vi "Test Timer Module API.vi"() -> ()   [LabVIEW 2018]
doc: "Timer Module API Tester."
uses:
  Timer Module.lvlib
panel:
  out "Timers":timestamp[](array[timestamp]) format="%^<%H:%M:%S%3u>T"
  in  "Pause Timer":bool
  in  "Start/Reset Timer":bool
  in  "Run as Singleton?":bool
  in  "Show Block Diagram":bool
  in  "Refresh Modules":bool
  out "Active Modules":string[](array[string])
  in  "Stop Module":bool
  in  "Select Module":i32(ring)=-1 caption="Select Module\nTo send Request to" items=["All"=-1]
  in  "Run New Module":bool
  in  "Hide Module Panel":bool
  in  "Show Module Panel":bool
  out "Status":string
  # "This VI tests the API for the Module."
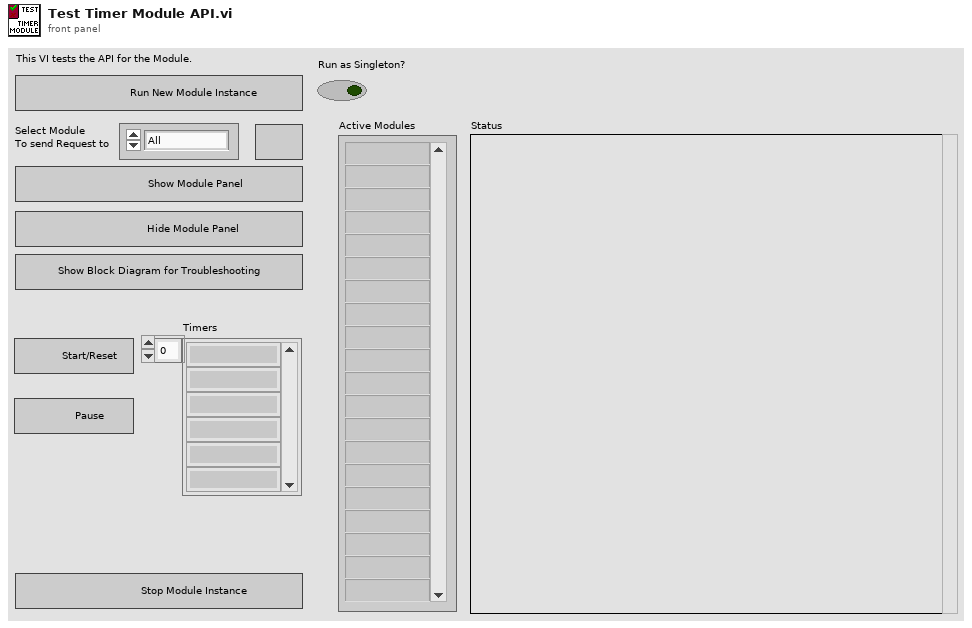
[diagram p1: front panel]
types:
  T1 = typedef "Timer Module.lvlib/Broadcast Events--cluster.ctl" = cluster{"Module Did Init":refnum<user-event>, "Status Updated":refnum<user-event>, "Error Reported":refnum<user-event>, "Module Did Stop":refnum<user-event>, "Update Module Execution Status":refnum<user-event>, "Timer Updated":refnum<user-event>}
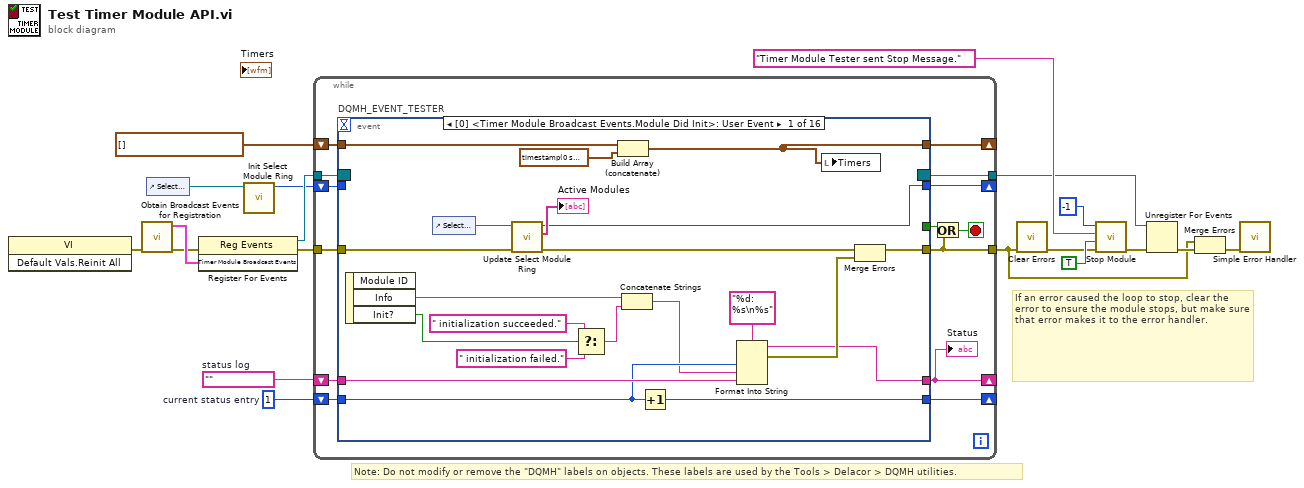
[diagram p0: block diagram]
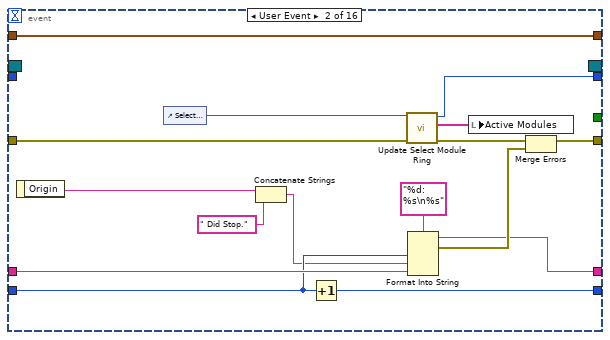
[diagram p2: hidden frame]
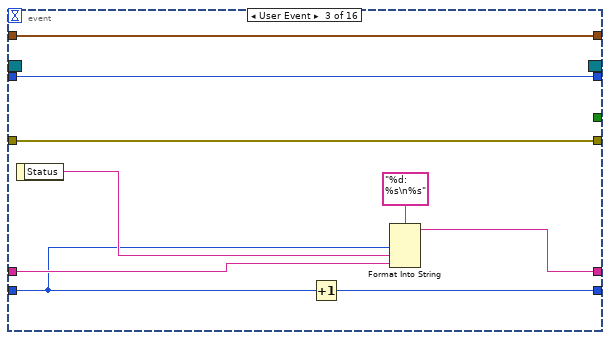
[diagram p3: hidden frame]
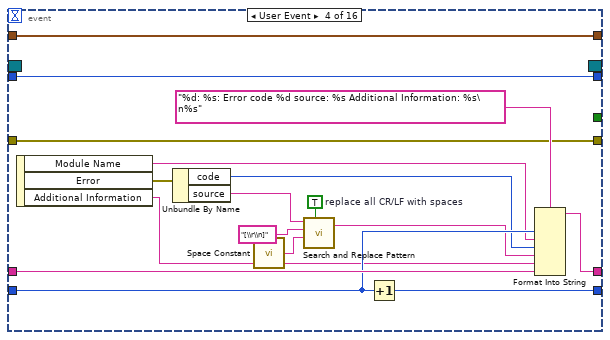
[diagram p4: hidden frame]
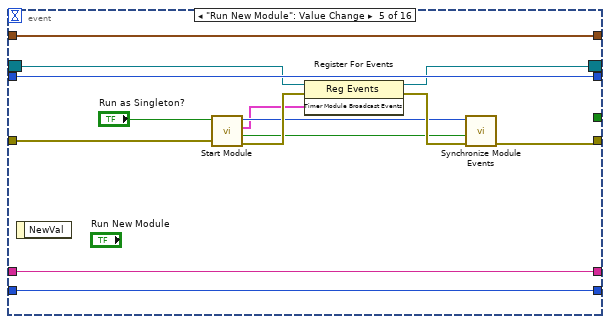
[diagram p5: hidden frame]
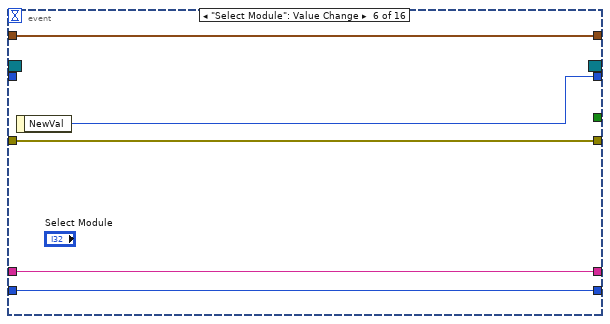
[diagram p6: hidden frame]
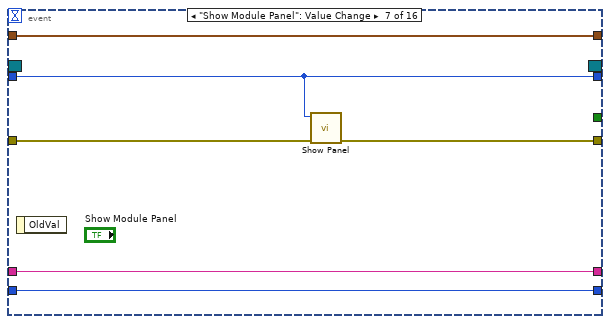
[diagram p7: hidden frame]
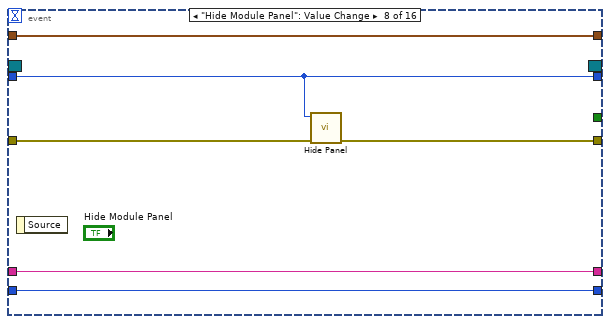
[diagram p8: hidden frame]
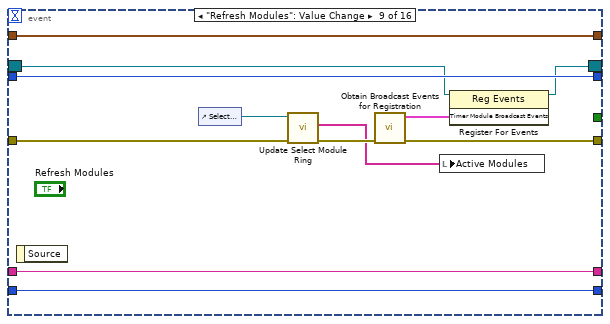
[diagram p9: hidden frame]
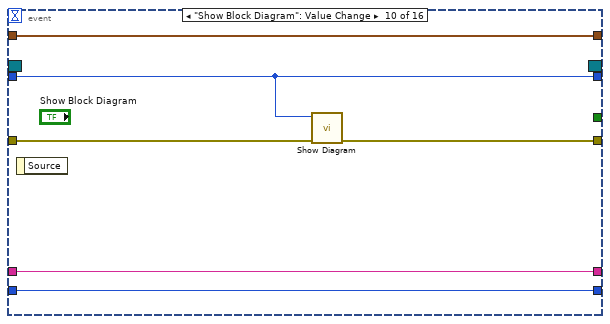
[diagram p10: hidden frame]
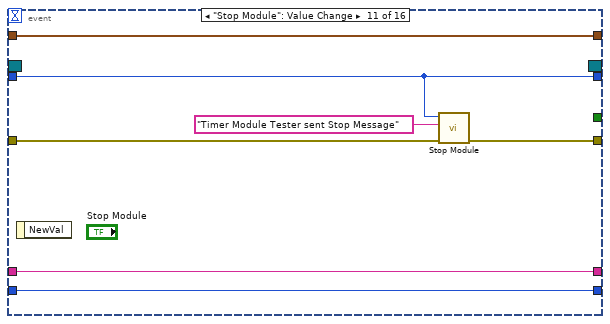
[diagram p11: hidden frame]
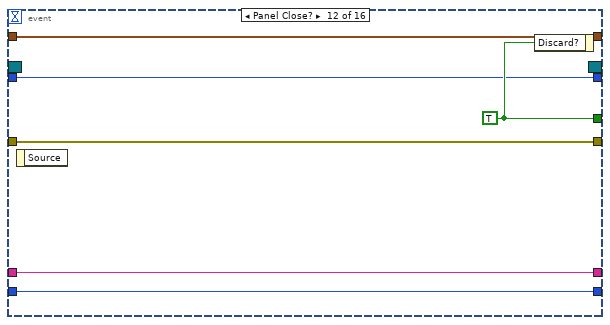
[diagram p12: hidden frame]
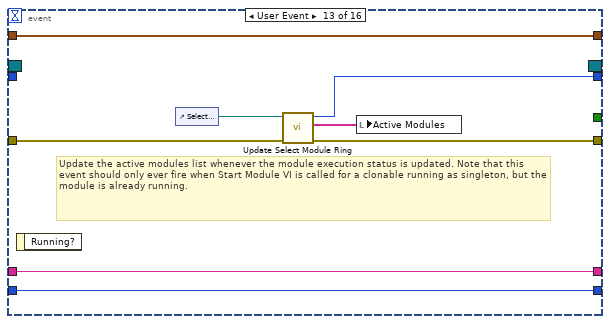
[diagram p13: hidden frame]
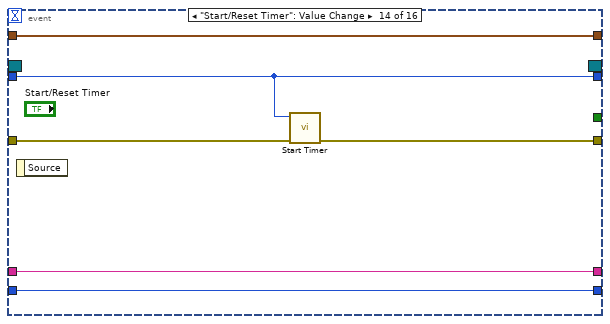
[diagram p14: hidden frame]
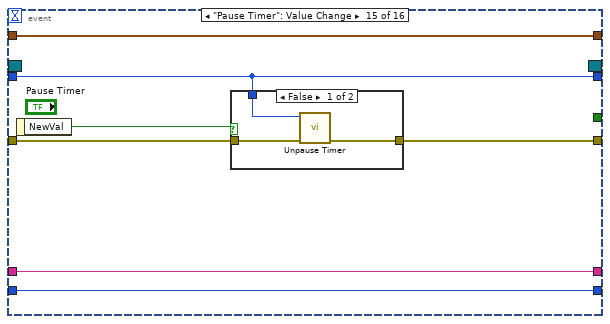
[diagram p15: hidden frame]
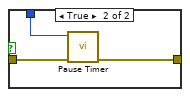
[diagram p16: hidden frame]
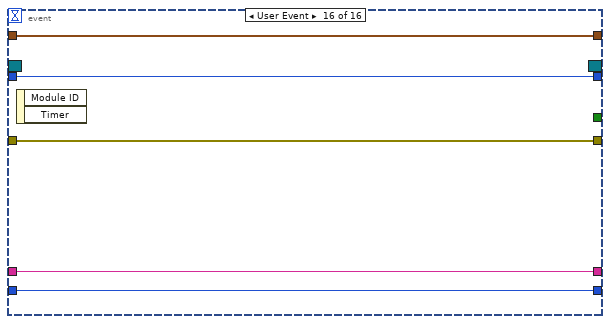
[diagram p17: hidden frame]
diagram:
  w15 = 1  # current status entry
  w16 = ""  # status log
  # "If an error caused the loop to stop, clear the error to ensure the module stops, but make sure that error makes it to the error handler."
  # "Note: Do not modify or remove the \"DQMH\" labels on objects. These labels are used by the Tools > Delacor > DQMH utilities."
  n1 = invoke class="VI" method="Default Vals.Reinit All"() -> (error out=w3:errorcluster)  [unwired: 3 in, 2 out]
  n2 = call "Obtain Broadcast Events for Registration.vi"("error in (no error)"=w3) -> ("error out"=w2:errorcluster, "Timer Module Broadcast Events"=w12:T1)  [unwired: 9 in]
  n3 = control-ref of="Select Module"() -> (w13:refnum<vi>)
  n4 = register-events(error in=w2, w12) -> (reference out=w19:refnum<event-registration>, error out=w11:errorcluster)  [unwired: 1 in]
  n5 = call "Init Select Module Ring.vi"("Select Module Ring Ref"=w13) -> ("Value for All Modules"=w14:i32)  [unwired: 8 in, 2 out]
  n6 = while {
    tunnel: w19 -> [w33]
    tunnel: [w22] -> w4
    tunnel: w11 -> [w31]
    shift-right: [w27] -> _
    shift-left: w16 -> [w29]
    shift-right: [w28] -> _
    shift-left: w15 -> [w30]
    shift-right: [w24] -> _
    shift-left: w14 -> [w25]
    tunnel: [w23] -> w8
    shift-right: [w20] -> _
    shift-left: timestamp[] [] ("Timers") -> [w21]
    stop <- w26 stop-if-true
    n7 = event "DQMH_EVENT_TESTER" shown="[0] <Timer Module Broadcast Events.Module Did Init>: User Event" {
      selector: w33 -> [_ _ _ _ w104 _ _ _ w134 _ _ _ _ _ _ _]
      dyn-events: [_ _ _ _ w103 _ _ _ w133 _ _ _ _ _ _ _] -> w23
      timeout: _ -> [_ _ _ _ _ _ _ _ _ _ _ _ _ _ _ _]
      tunnel: [_ _ _ _ _ _ _ _ _ _ _ w158 _ _ _ _] -> w32
      tunnel: [w44 w62 w79 w86 w102 w115 w120 w126 w130 w142 w148 w157 w162 w169 w176 w190] -> w22
      tunnel: w31 -> [w46 w64 w79 w86 w105 w115 w121 w127 w135 w145 w149 w157 w163 w172 w179 w190]
      tunnel: w30 -> [w51 w67 w72 w92 w107 w113 w118 w124 w138 w143 w151 w155 w165 w170 w177 w188]
      tunnel: w29 -> [w52 w68 w75 w94 w108 w114 w119 w125 w139 w144 w152 w156 w166 w171 w178 w189]
      tunnel: [w49 w65 w76 w89 w108 w114 w119 w125 w139 w144 w152 w156 w166 w171 w178 w189] -> w27
      tunnel: [w50 w66 w78 w95 w107 w113 w118 w124 w138 w143 w151 w155 w165 w170 w177 w188] -> w28
      tunnel: w25 -> [_ _ w73 w96 w106 _ w117 w123 w137 w141 w150 w154 _ w168 w175 w187]
      tunnel: [w41 w59 w73 w96 w106 w112 w117 w123 w137 w141 w150 w154 w161 w168 w175 w187] -> w24
      tunnel: w21 -> [w36 w55 w71 w80 w97 w111 w116 w122 w128 w140 w146 w153 w159 w167 w173 w186]
      tunnel: [w34 w55 w71 w80 w97 w111 w116 w122 w128 w140 w146 w153 w159 w167 w173 w186] -> w20
      event User Event {
        n8 = event-data() -> ("Info"=w48:string, "Init?"=w38:bool)  [unwired: 1 in, 1 out]
        n9 = control-ref of="Select Module"() -> (w43:refnum<vi>)
        n10 = call "Update Select Module Ring.vi"("error in (no error)"=w46, "Select Module Ring Ref"=w43) -> ("error out"=w45:errorcluster, "Active Modules (Array)"=→"Active Modules":string[], "New Module Ring Value"=w41:i32)  [unwired: 7 in]
        n11 = Select(t=" initialization succeeded.", s=w38, f=" initialization failed.") -> (s? t:f=w37:string)
        n12 = Build Array (concatenate)(w36, timestamp(0 s since 1904-01-01) ("Timer")) -> (w34:timestamp[])
        n13 = Concatenate Strings(w48, w37) -> (w47:string)
        n14 = Increment(x=w51) -> (x+1=w50:i32)
        n15 = Format Into String(format string="%d: %s\n%s", w51, w47, w52) -> (resulting string=w49:string, error out=w54:errorcluster)  [unwired: 2 in]
        n16 = local write "Timers"(w34) -> ()
        n17 = Merge Errors(w45, w54) -> (w44:errorcluster)
      }
      event User Event {
        n18 = event-data() -> ("Origin"=w57:string)  [unwired: 1 in]
        n19 = control-ref of="Select Module"() -> (w61:refnum<vi>)
        n20 = Concatenate Strings(w57, " Did Stop.") -> (w56:string)
        n21 = Increment(x=w67) -> (x+1=w66:i32)
        n22 = call "Update Select Module Ring.vi"("error in (no error)"=w64, "Select Module Ring Ref"=w61) -> ("error out"=w63:errorcluster, "Active Modules (Array)"=w60:string[], "New Module Ring Value"=w59:i32)  [unwired: 7 in]
        n23 = Format Into String(format string="%d: %s\n%s", w67, w56, w68) -> (resulting string=w65:string, error out=w70:errorcluster)  [unwired: 2 in]
        n24 = local write "Active Modules"(w60) -> ()
        n25 = Merge Errors(w63, w70) -> (w62:errorcluster)
      }
      event User Event {
        n26 = event-data() -> ("Status"=w74:string)  [unwired: 1 in]
        n27 = Increment(x=w72) -> (x+1=w78:i32)
        n28 = Format Into String(format string="%d: %s\n%s", w72, w74, w75) -> (resulting string=w76:string)  [unwired: 2 in, 1 out]
      }
      event User Event {
        w90 = TRUE  # replace all CR/LF with spaces
        n29 = event-data() -> ("Module Name"=w84:string, "Error"=w83:errorcluster, "Additional Information"=w81:string)  [unwired: 1 in]
        n30 = Unbundle By Name(w83) -> ("code"=w85:i32, "source"=w87:string)
        n31 = call <vilib>:"Space Constant.vi"() -> ("String"=w91:string)
        n32 = call <vilib>:"Search and Replace Pattern.vi"("string"=w87, "regular expression (\"\")"="[\\r\\n]" ("regular expression (\"\")"), "replace string (\"\")"=w91, "replace all? (F)"=w90) -> ("result string"=w88:string)  [unwired: 1 in, 1 out]
        n33 = Increment(x=w92) -> (x+1=w95:i32)
        n34 = Format Into String(format string="%d: %s: Error code %d source: %s Additional Information: %s\n%s", w92, w84, w85, w88, w81, w94) -> (resulting string=w89:string)  [unwired: 2 in, 1 out]
      }
      event "Run New Module": Value Change {
        n35 = event-data() -> ()  [unwired: 1 in, 1 out]
        n36 = call "Start Module.vi"("error in (no error)"=w105, "Run as Singleton? (F)"="Run as Singleton?") -> ("error out"=w109:errorcluster, "Wait for Event Sync?"=w100:bool, "Timer Module Broadcast Events"=w99:T1, "Module ID"=w101:i32)  [unwired: 6 in]
        n37 = register-events(reference=w104, error in=w109, w99) -> (reference out=w103:refnum<event-registration>, error out=w110:errorcluster)
        n38 = call "Synchronize Module Events.vi"("error in (no error)"=w110, "Wait for Event Sync?"=w100, "Module ID"=w101) -> ("error out"=w102:errorcluster)  [unwired: 7 in, 1 out]
      }
      event "Select Module": Value Change {
        n39 = event-data() -> ("NewVal"=w112:i32)  [unwired: 1 in]
      }
      event "Show Module Panel": Value Change {
        n40 = event-data() -> ()  [unwired: 1 in, 1 out]
        n41 = call "Show Panel.vi"("error in (no error)"=w121, "Module ID"=w117) -> ("error out"=w120:errorcluster)  [unwired: 9 in]
      }
      event "Hide Module Panel": Value Change {
        n42 = event-data() -> ()  [unwired: 1 in, 1 out]
        n43 = call "Hide Panel.vi"("error in (no error)"=w127, "Module ID"=w123) -> ("error out"=w126:errorcluster)  [unwired: 9 in]
      }
      event "Refresh Modules": Value Change {
        n44 = event-data() -> ()  [unwired: 1 in, 1 out]
        n45 = control-ref of="Select Module"() -> (w136:refnum<vi>)
        n46 = call "Update Select Module Ring.vi"("error in (no error)"=w135, "Select Module Ring Ref"=w136) -> ("error out"=w131:errorcluster, "Active Modules (Array)"=w129:string[])  [unwired: 7 in, 1 out]
        n47 = call "Obtain Broadcast Events for Registration.vi"("error in (no error)"=w131) -> ("error out"=w130:errorcluster, "Timer Module Broadcast Events"=w132:T1)  [unwired: 9 in]
        n48 = local write "Active Modules"(w129) -> ()
        n49 = register-events(reference=w134, w132) -> (reference out=w133:refnum<event-registration>)  [unwired: 1 in, 1 out]
      }
      event "Show Block Diagram": Value Change {
        n50 = event-data() -> ()  [unwired: 1 in, 1 out]
        n51 = call "Show Diagram.vi"("error in (no error)"=w145, "Module ID"=w141) -> ("error out"=w142:errorcluster)  [unwired: 9 in]
      }
      event "Stop Module": Value Change {
        n52 = event-data() -> ()  [unwired: 1 in, 1 out]
        n53 = call "Stop Module.vi"("error in (no error)"=w149, "Origin"="Timer Module Tester sent Stop Message", "Module ID"=w150) -> ("error out"=w148:errorcluster)  [unwired: 8 in]
      }
      event Panel Close? {
        w158 = TRUE ("Discard?")
        n54 = event-data() -> ()  [unwired: 1 in, 1 out]
        n55 = event-data("Discard?"=w158) -> ()  [unwired: 1 in, 1 out]
      }
      event User Event {
        # "Update the active modules list whenever the module execution status is updated. Note that this event should only ever fire when Start Module VI is called for a clonable running as singleton, but the module is already running."
        n56 = event-data() -> ()  [unwired: 1 in, 1 out]
        n57 = control-ref of="Select Module"() -> (w164:refnum<vi>)
        n58 = call "Update Select Module Ring.vi"("error in (no error)"=w163, "Select Module Ring Ref"=w164) -> ("error out"=w162:errorcluster, "Active Modules (Array)"=w160:string[], "New Module Ring Value"=w161:i32)  [unwired: 7 in]
        n59 = local write "Active Modules"(w160) -> ()
      }
      event "Start/Reset Timer": Value Change {
        n60 = event-data() -> ()  [unwired: 1 in, 1 out]
        n61 = call "Start Timer.vi"("error in (no error)"=w172, "Module ID"=w168) -> ("error out"=w169:errorcluster)  [unwired: 9 in]
      }
      event "Pause Timer": Value Change {
        n62 = event-data() -> ("NewVal"=w174:bool)  [unwired: 1 in]
        n63 = case shown="False" w174 {
          tunnel: w179 -> [w182 w185]
          tunnel: [w181 w184] -> w176
          tunnel: w175 -> [w180 w183]
          frame False {
            n64 = call "Unpause Timer.vi"("error in (no error)"=w182, "Module ID"=w180) -> ("error out"=w181:errorcluster)  [unwired: 9 in]
          }
          frame True {
            n65 = call "Pause Timer.vi"("error in (no error)"=w185, "Module ID"=w183) -> ("error out"=w184:errorcluster)  [unwired: 9 in]
          }
        }
      }
      event User Event {
        n66 = event-data() -> ()  [unwired: 1 in, 2 out]
      }
    }
    "Status" <- w27
    n67 = Or(x=w32, y=w22) -> (x .or. y?=w26:bool)
  }
  n68 = call <vilib>:"Clear Errors.vi"("error in (no error)"=w4) -> ("error out"=w6:errorcluster)  [unwired: 5 in, 1 out]
  n69 = call "Stop Module.vi"("error in (no error)"=w6, "Wait for Module to stop? (F)"=TRUE ("Wait for Module to stop?"), "Origin"="Timer Module Tester sent Stop Message.", "Module ID"=-1 ("Stop all")) -> ("error out"=w17:errorcluster)  [unwired: 7 in]
  n70 = Unregister For Events(event registration refnum=w8, error in=w17) -> (error out=w18:errorcluster)
  n71 = Merge Errors(w4, w18) -> (w5:errorcluster)
  n72 = call <vilib>:"Simple Error Handler.vi"("error in (no error)"=w5) -> ()  [unwired: 4 in, 5 out]
